vi "Add VI or CTL to Virtual Folder.vi"(4 "Virtual Folder Type":T1, 6 "Virtual Folder Search Results":T2, 8 "error in":errorcluster, 10 "VI Ref":refnum<vi>, 11 "lvlib or lvclass Ref":refnum<vi>) -> (0 "error out":errorcluster)   [LabVIEW 2022 SP3]
doc: "This VI adds the newly created VI or CTL to a virtual folder.\n\nThis VI assumes that the newly created VI has already been saved to disk (i.e. already exists on disk)."
uses:
  DFS Output (cluster).ctl
  Virtual Folder Type (enum).ctl
panel:
  # "Development\ncontrols/indicators useful for development and testing, but which are not outputs of the VI"
  # "Input\nInputs to the VI"
  # "Output\nOutputs of the VI"
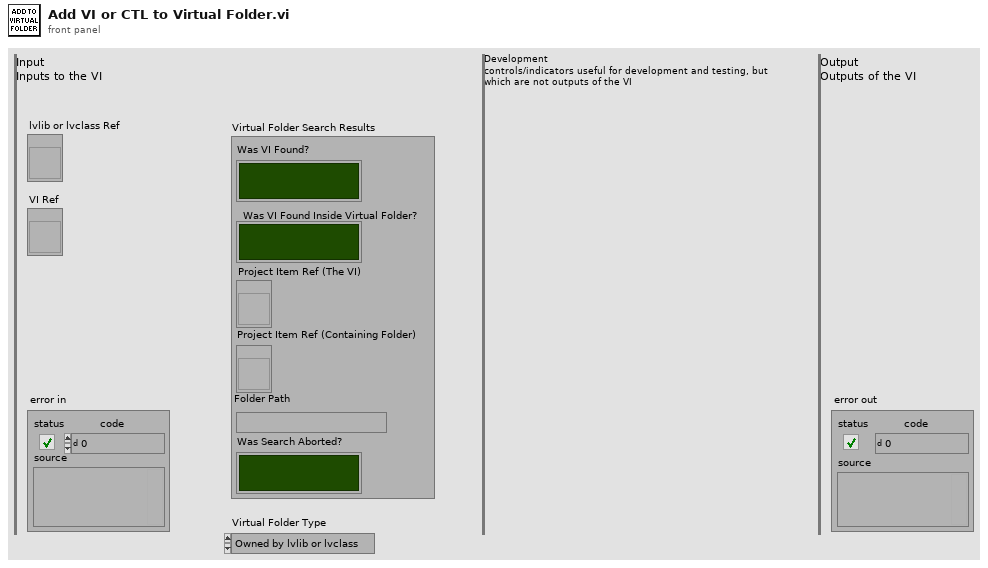
[diagram p1: front panel]
types:
  T1 = typedef "Virtual Folder Type (enum).ctl" = enum16{"Owned by lvlib or lvclass", "Owned by lvproj"}
  T2 = typedef "DFS Output (cluster).ctl" = cluster{"Was VI Found?":bool, "Was VI Found Inside Virtual Folder?":bool, "Project Item Ref (The VI)":refnum<vi>, "Project Item Ref (Containing Folder)":refnum<vi>, "Folder Path":string, "Was Search Aborted?":bool}
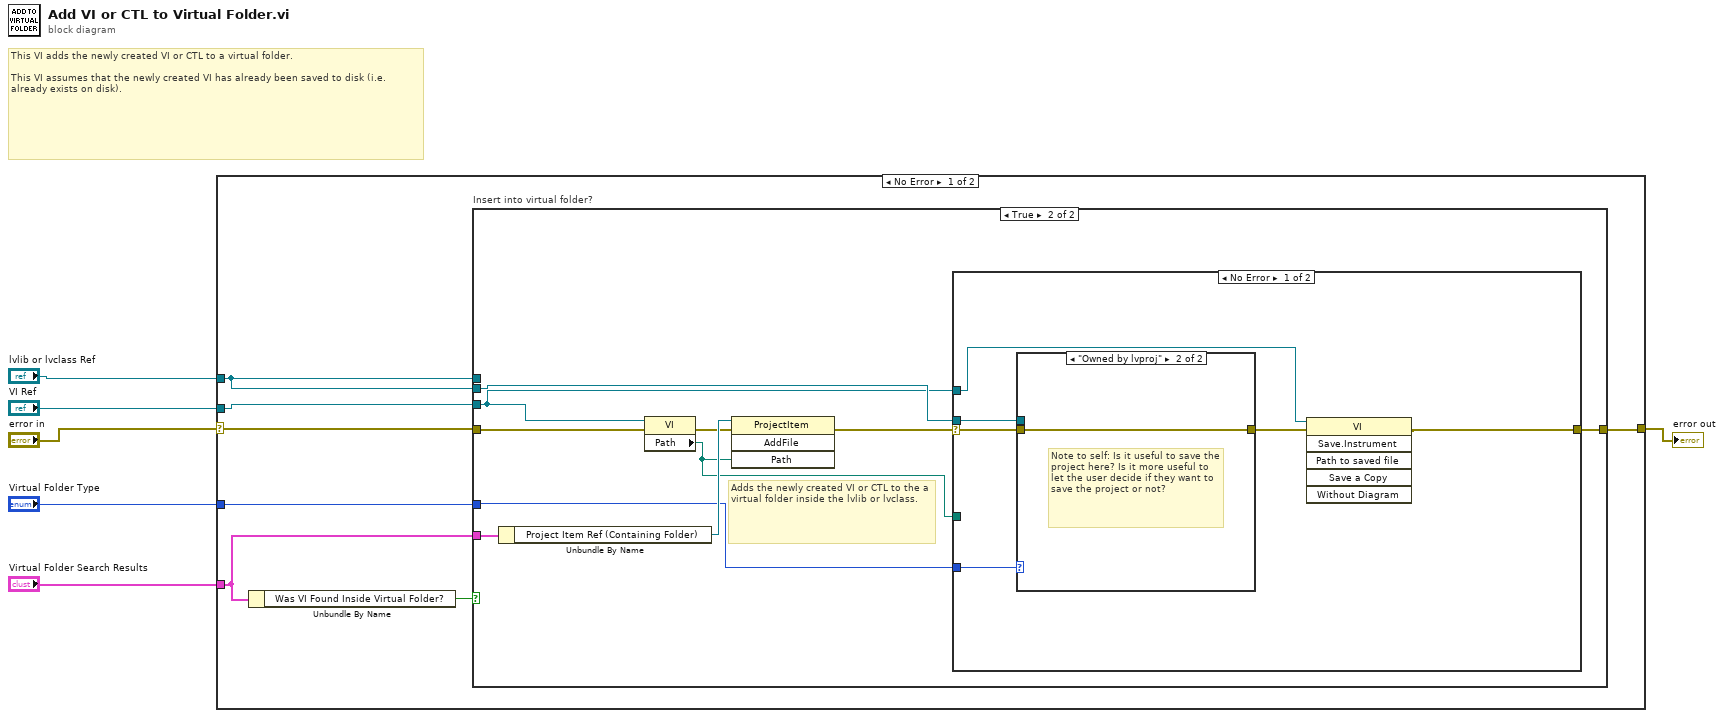
[diagram p0: block diagram]
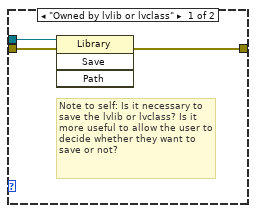
[diagram p3: hidden frame]
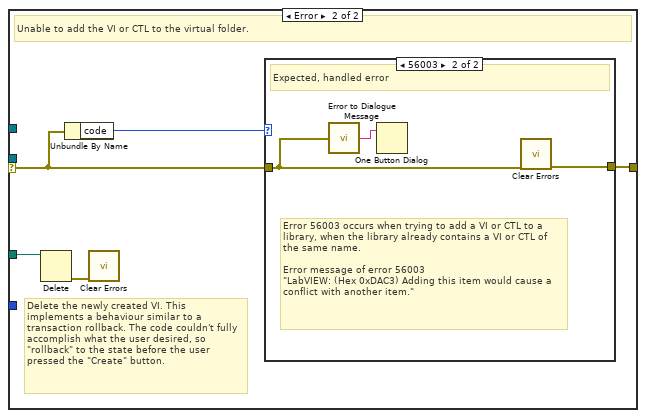
[diagram p4: hidden frame]
diagram:
  # "This VI adds the newly created VI or CTL to a virtual folder.\n\nThis VI assumes that the newly created VI has already been saved to disk (i.e. already exists on disk)."
  n1 = case shown="No Error" "error in" {
    selector: "error in" -> [w10 w44]
    tunnel: [w7 w44] -> w5
    tunnel: "lvlib or lvclass Ref" -> [w9 _]
    tunnel: "VI Ref" -> [w11 _]
    tunnel: "Virtual Folder Search Results" -> [w12 _]
    tunnel: "Virtual Folder Type" -> [w8 _]
    frame No Error {
      n2 = Unbundle By Name(w12) -> ("Was VI Found Inside Virtual Folder?"=w13:bool)
      n3 = case "Insert into virtual folder?" shown="True" w13 {
        tunnel: w9 -> [_ _]
        tunnel: [w14 w18] -> w7
        tunnel: w12 -> [_ w24]
        tunnel: w11 -> [_ w19]
        tunnel: w10 -> [w14 w22]
        tunnel: w9 -> [_ w20]
        tunnel: w8 -> [_ w15]
        frame False {
        }
        frame True {
          # "Adds the newly created VI or CTL to the a virtual folder inside the lvlib or lvclass."
          n4 = Unbundle By Name(w24) -> ("Project Item Ref (Containing Folder)"=w23:refnum<vi>)
          n5 = property class="VI"(reference=w19, error in=w22) -> (error out=w21:errorcluster, "Path"=w16:path)  [unwired: 1 out]
          n6 = invoke class="ProjectItem" method="AddFile"(reference=w23, error in=w21, "Path"=w16) -> (error out=w17:errorcluster)  [unwired: 1 in, 3 out]
          n7 = case shown="No Error" w17 {
            selector: w17 -> [w30 w37]
            tunnel: w20 -> [w28 _]
            tunnel: [w27 w38] -> w18
            tunnel: w19 -> [w26 _]
            tunnel: w16 -> [_ w36]
            tunnel: w15 -> [w25 _]
            frame No Error {
              n8 = case shown="\"Owned by lvproj\"" w25 {
                tunnel: w30 -> [w33 w34]
                tunnel: [w32 w34] -> w29
                tunnel: w28 -> [w31 _]
                frame "Owned by lvlib or lvclass" {
                  # "Note to self: Is it necessary to save the lvlib or lvclass? Is it more useful to allow the user to decide whether they want to save or not?"
                  n9 = invoke class="Library" method="Save"(reference=w31, error in=w33) -> (error out=w32:errorcluster)  [unwired: 2 in, 3 out]
                }
                frame "Owned by lvproj" {
                  # "Note to self: Is it useful to save the project here? Is it more useful to let the user decide if they want to save the project or not?"
                }
              }
              n10 = invoke class="VI" method="Save.Instrument"(reference=w26, error in=w29) -> (error out=w27:errorcluster)  [unwired: 4 in, 5 out]
            }
            frame Error {
              # "Delete the newly created VI. This implements a behaviour similar to a transaction rollback. The code couldn't fully accomplish what the user desired, so \"rollback\" to the state before the user pressed the \"Create\" button."
              # "Unable to add the VI or CTL to the virtual folder."
              n11 = Delete(path (use dialog)=w36) -> (error out=w35:errorcluster)  [unwired: 4 in, 2 out]
              n12 = Unbundle By Name(w37) -> ("code"=w39:i32)
              n13 = call <vilib>:"Clear Errors.vi"("error in (no error)"=w35) -> ()  [unwired: 5 in, 2 out]
              n14 = case shown="56003" w39 {
                tunnel: w37 -> [w40 w42]
                tunnel: [w40 w43] -> w38
                frame Default {
                  # "Do nothing. The error will be handled downstream."
                  # "Unexpected error"
                }
                frame 56003 {
                  # "Error 56003 occurs when trying to add a VI or CTL to a library, when the library already contains a VI or CTL of the same name.\n\nError message of error 56003\n\"LabVIEW: (Hex 0xDAC3) Adding this item would cause a conflict with another item.\""
                  # "Expected, handled error"
                  n15 = call "Error to Dialogue Message.vi"("error in"=w42) -> ("Dialogue Message"=w41:string)
                  n16 = One Button Dialog(message=w41) -> ()  [unwired: 1 in, 1 out]
                  n17 = call <vilib>:"Clear Errors.vi"("error in (no error)"=w42) -> ("error out"=w43:errorcluster)  [unwired: 5 in, 1 out]
                }
              }
            }
          }
        }
      }
    }
    frame Error {
    }
  }
  "error out" <- w5
